vi "getParameters.vi"(11 "ClearAOSCorrectionCommand in":refnum<class "ClearAOSCorrectionCommand.lvclass">) -> (2 "Parameters":T1, 3 "ClearAOSCorrectionCommand out":refnum<class "ClearAOSCorrectionCommand.lvclass">)   [LabVIEW 2016, in "ClearAOSCorrectionCommand.lvclass"]
uses:
  ClearAOSCorrectionCommand.lvclass
  DataTypes/Topics/CommandClearAOSCorrection.ctl
  DataTypes/Topics/Parts/CommandId.ctl
  ClearAOSCorrectionCommand.lvclass/ClearAOSCorrectionCommand.ctl
  DataTypes/Topics/M1M3SupportTopics.lvlib
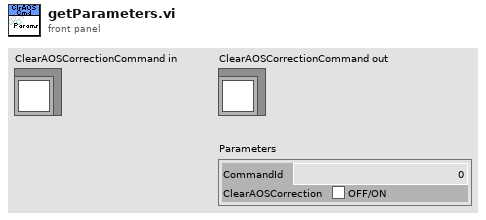
[diagram p1: front panel]
types:
  T1 = typedef "M1M3SupportTopics.lvlib/CommandClearAOSCorrection.ctl" = cluster{"CommandId":T2, "ClearAOSCorrection":bool}
  T2 = typedef "M1M3SupportTopics.lvlib/CommandId.ctl" = i32
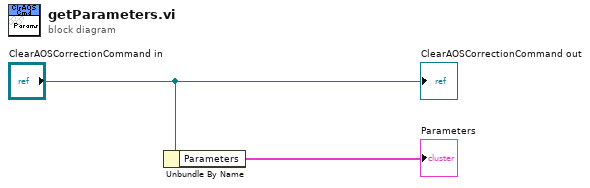
[diagram p0: block diagram]
diagram:
  n1 = Unbundle By Name("ClearAOSCorrectionCommand in") -> ("Parameters"=→"Parameters":T1)
  "ClearAOSCorrectionCommand out" <- "ClearAOSCorrectionCommand in"
